vi "MAIN.vi"() -> ()   [LabVIEW 2017]
uses:
  Typedefs/Instructions.ctl
  Typedefs/State Information.ctl
  <vilib>/Utility/error.llb/DialogType.ctl
  Typedefs/Temperature Profile.ctl
  Typedefs/Status.ctl
  <vilib>/event_ctls.llb/usereventprio.ctl
  <vilib>/DAQmx/read.llb/DAQmx Read (Analog Wfm 1Chan NSamp).vi
  <vilib>/DAQmx/miscellaneous.llb/DAQmx Fill In Error Info.vi
  <vilib>/Utility/file.llb/Write To Spreadsheet File (DBL).vi
  <resource>/objmgr/daqmx.rc
panel:
  in  "Tab Control":enum32{"Settings", "Charts"}(tab)
  in  "Linkam Controller":refnum<visa-resource-name>="COM1"
  in  "Temp loop delay":u32=100
  out "Current Temperature Loop Error":errorcluster
  in  "physical channels":tag="Dev1/ai0"
  out "Slide":i32(slide) scale=15.0..1.0
  out "Voltage":waveform(dbl)(graph)
  out "Temperature":dbl(graph)
  in  "Temperature Profile":dbl[][](array[numeric])=[[20.0, 0.0], [1.0, -30.0]]
  out "Status":string
  out "Error":string
  out "Pump":u8
  out "°C":dbl
  in  "Start":bool
  in  "Hold":bool
  in  "Stop":bool
  in  "Disconnect":bool
  out "Current Ramp":i32
  out "Time (ms)":i32
  out "Loop 2 Timer":u32
  out "Loop 1 Timer":u32
  in  "Rate":dbl=1000.0 format="%0.2f"
  out "Samples":i32
  # "Rate(°C/min)"
  # "Hold (s)"
  # "Limit (°C)"
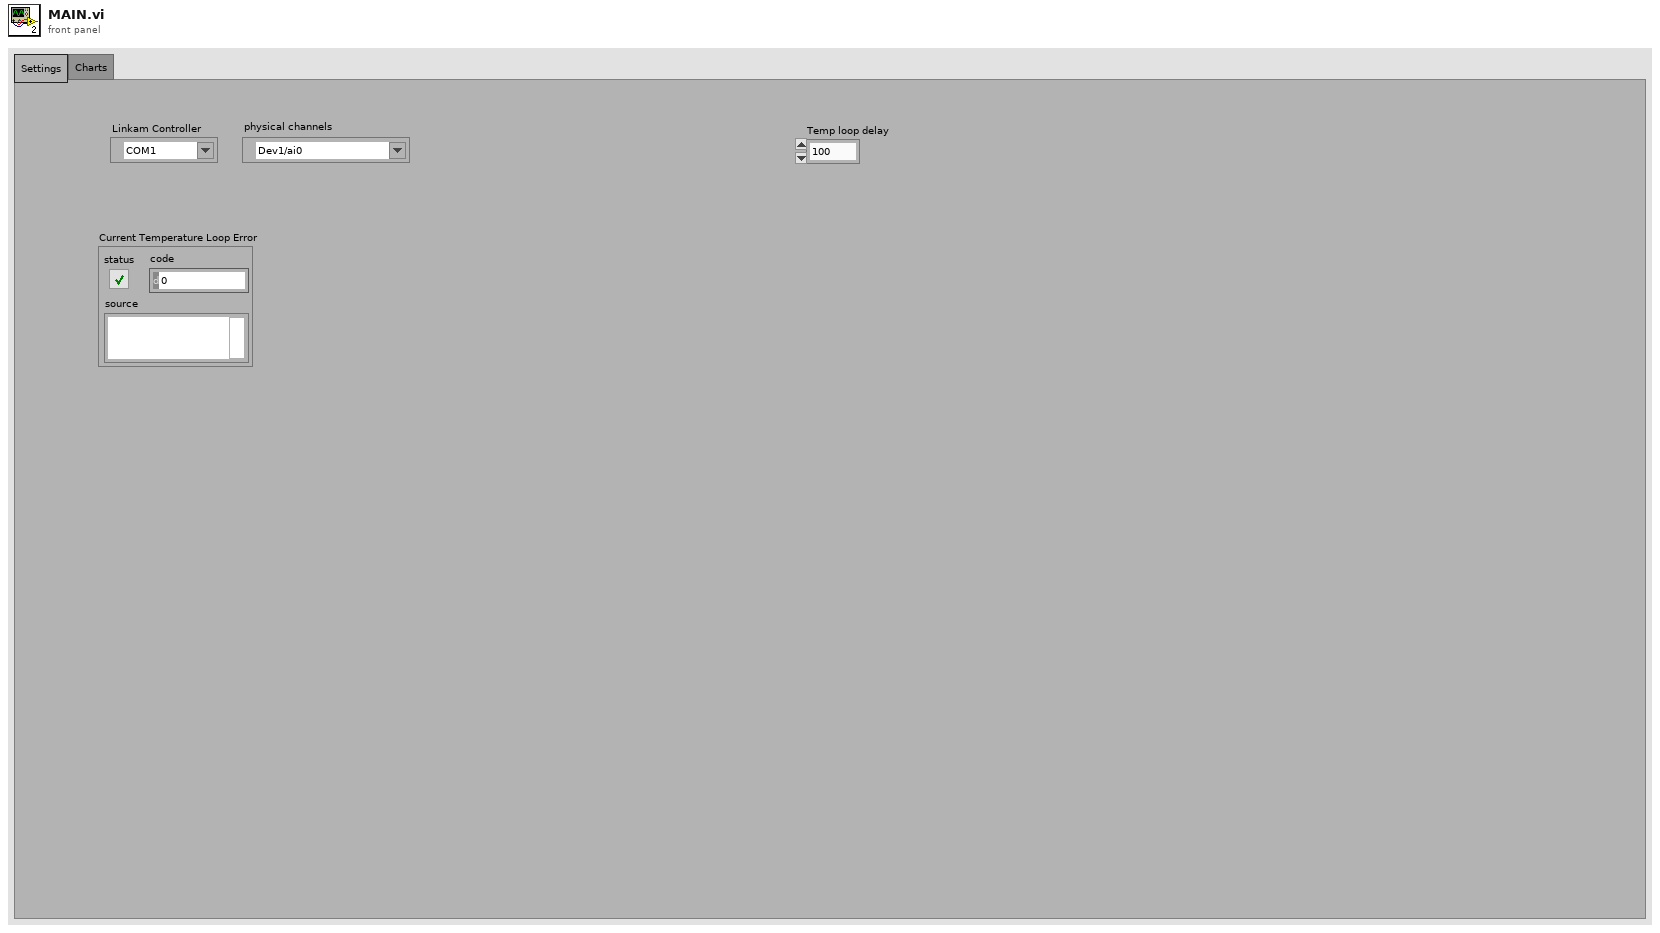
[diagram p1: front panel]
types:
  T1 = typedef "DialogType.ctl" = u16
  T2 = typedef "State Information.ctl" = cluster{"Ramp":i32, "Total Ramp":i32, "Time":i32, "Total Time":i32, "Start Time":dbl}
  T3 = typedef "Instructions.ctl" = enum16{"Idle", "Start", "Get Profile", "Go to Limit", "Hold Limit Time", "Stop", "Disconnect"}
  T4 = typedef "Temperature Profile.ctl" = enum16{"Rate", "Limit", "Hold Time"}
  T5 = typedef "Status.ctl" = enum16{"No Status", "Stopped", "Heating", "Cooling", "Limit Reached", "Holding the Limit Time", "Manual Hold"}
  T6 = typedef "usereventprio.ctl" = enum32{"high priority", "normal priority"}
  T7 = cluster{"Temperature":dbl, "Status":string, "Error":string, "Pump":u8}
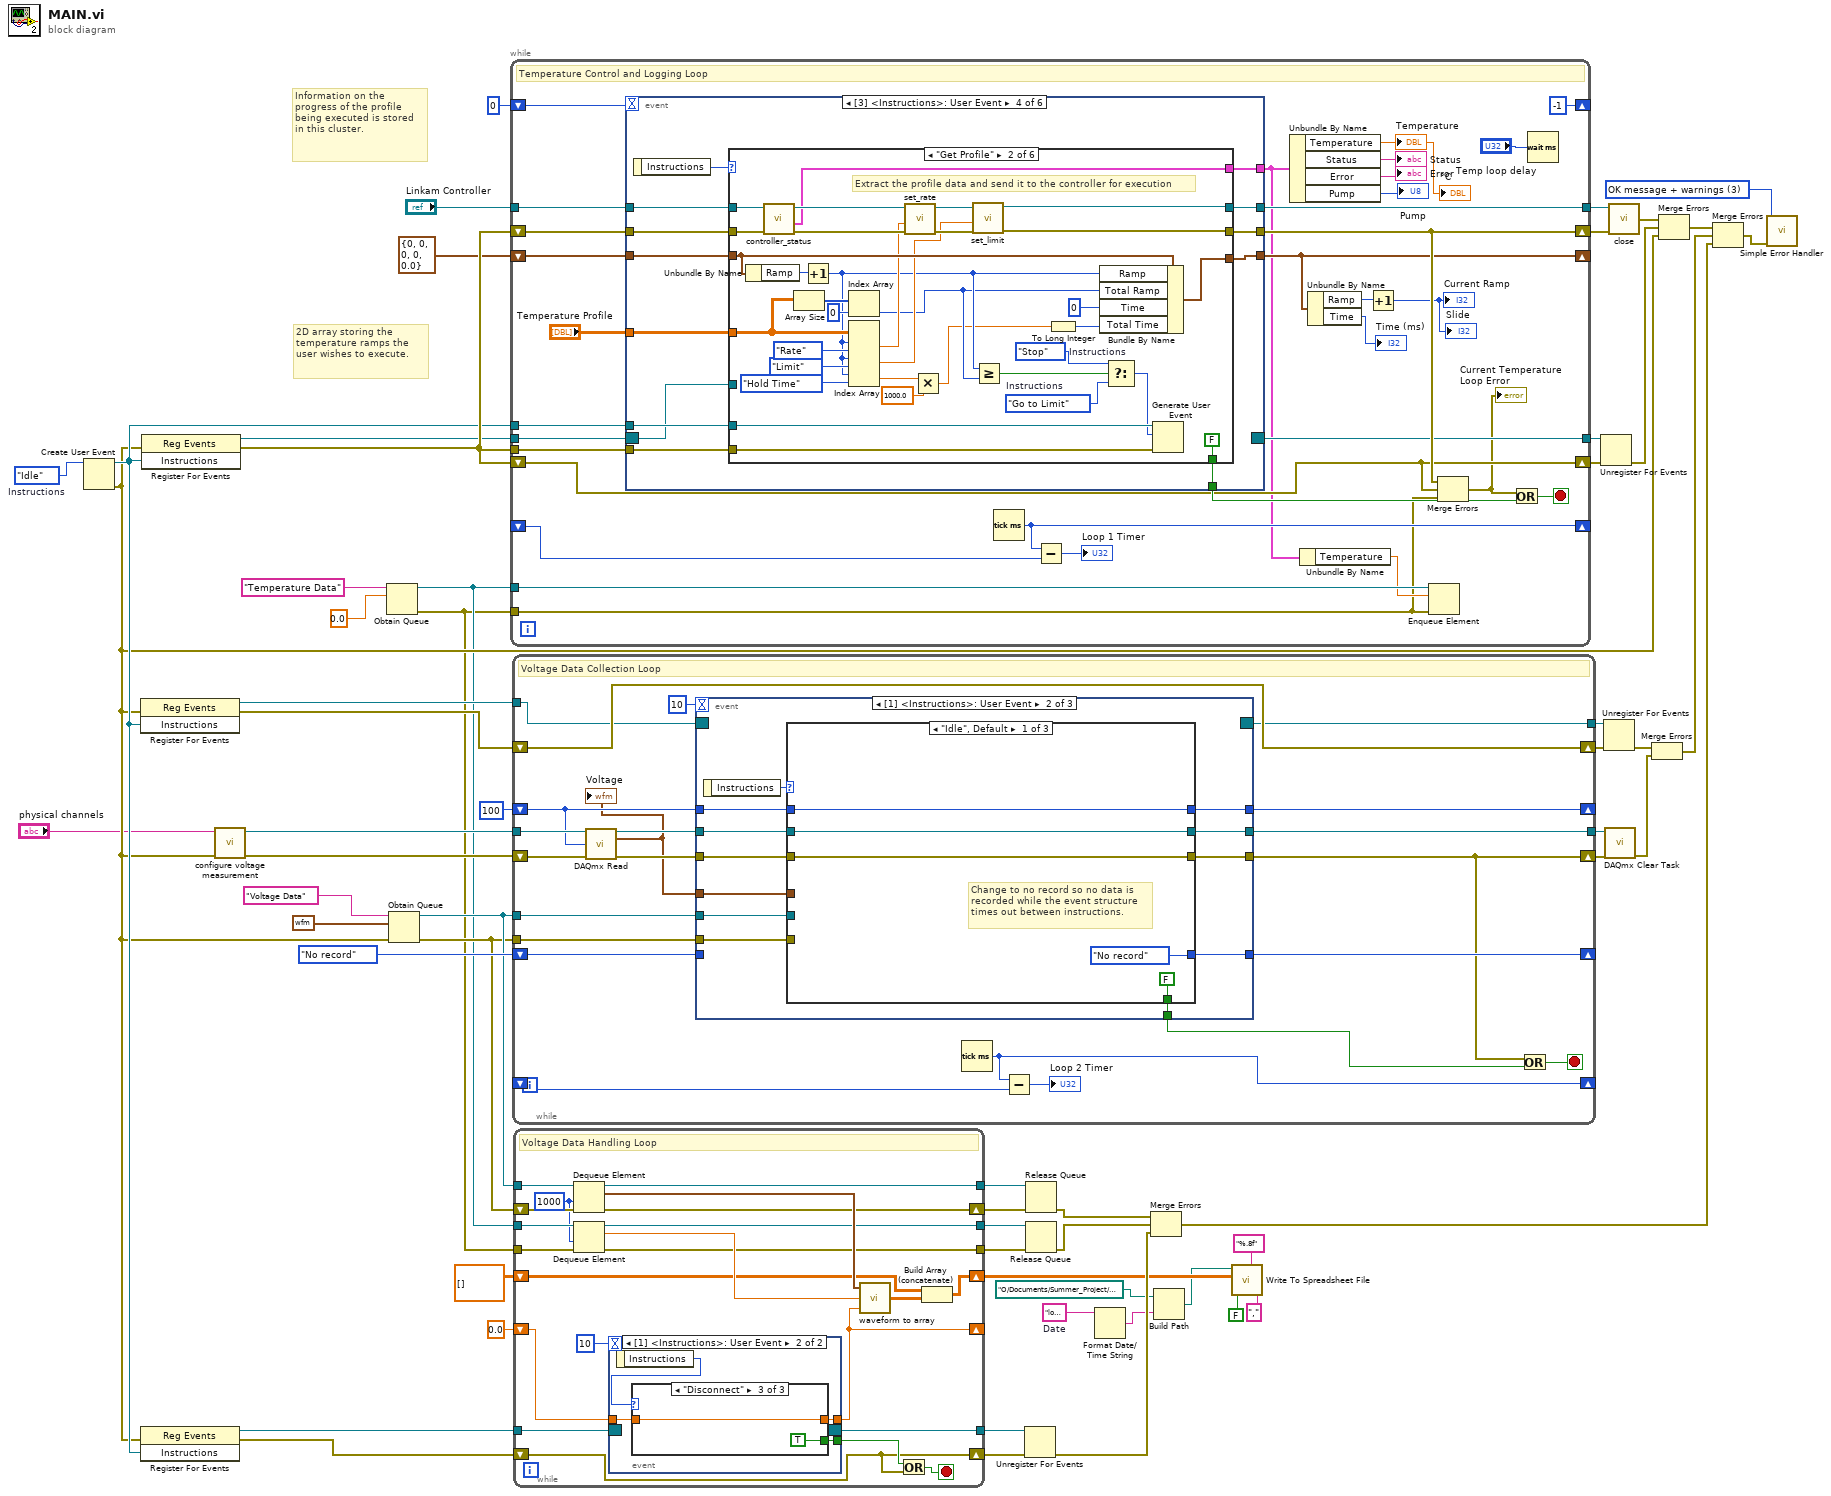
[diagram p0: block diagram]
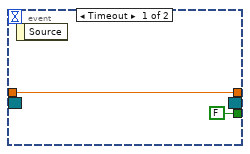
[diagram p2: hidden frame]
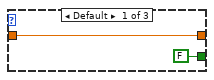
[diagram p3: hidden frame]
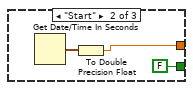
[diagram p4: hidden frame]
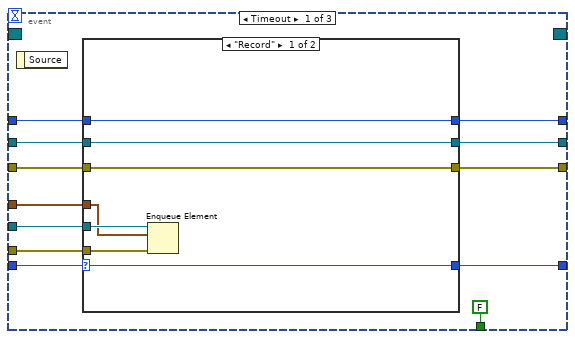
[diagram p5: hidden frame]
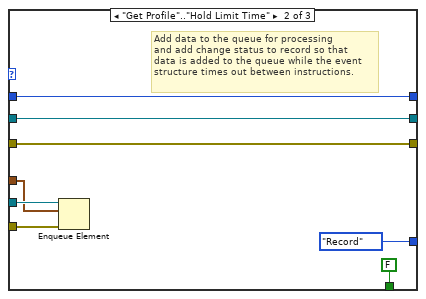
[diagram p7: hidden frame]
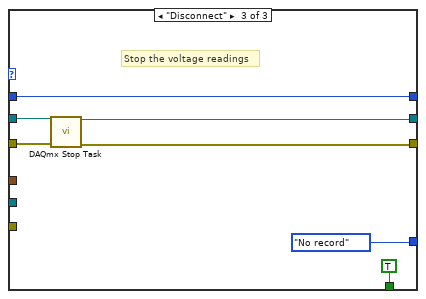
[diagram p8: hidden frame]
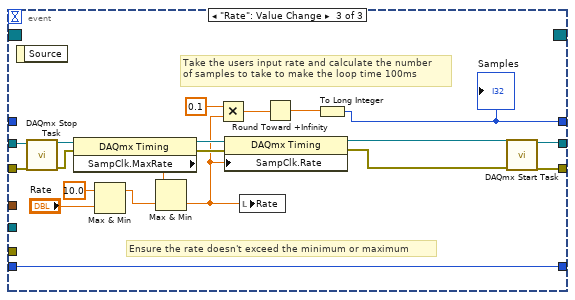
[diagram p9: hidden frame]
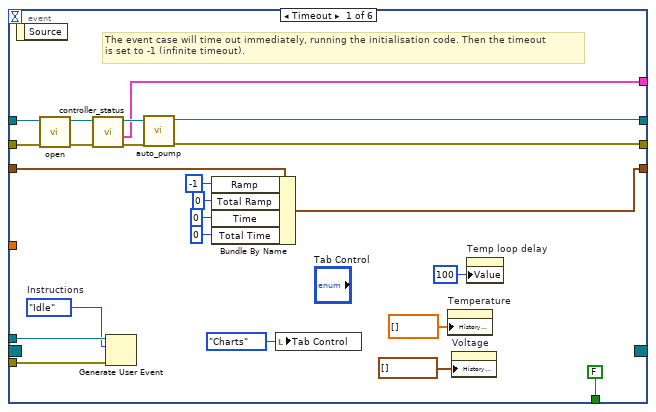
[diagram p10: hidden frame]
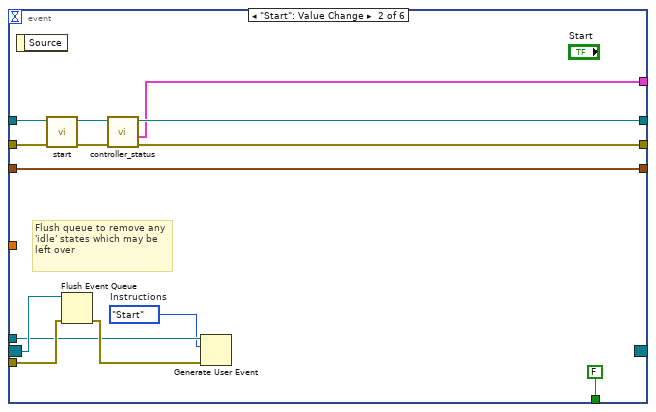
[diagram p11: hidden frame]
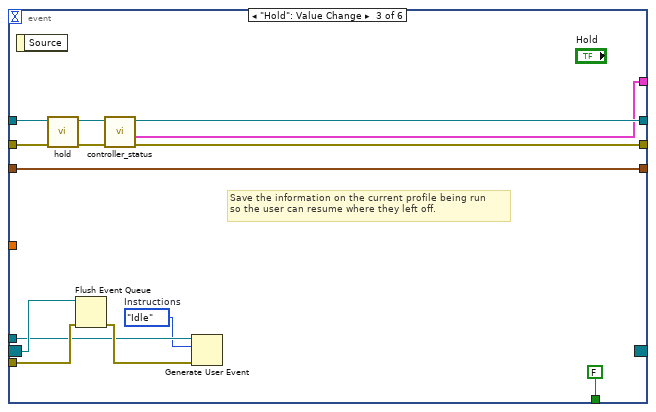
[diagram p12: hidden frame]
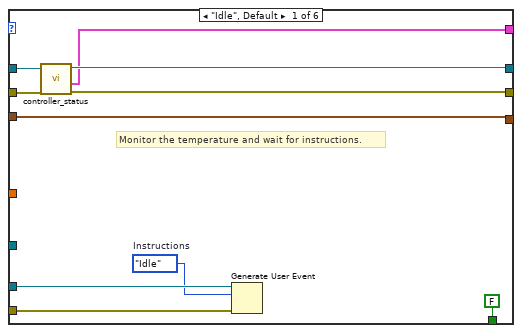
[diagram p13: hidden frame]
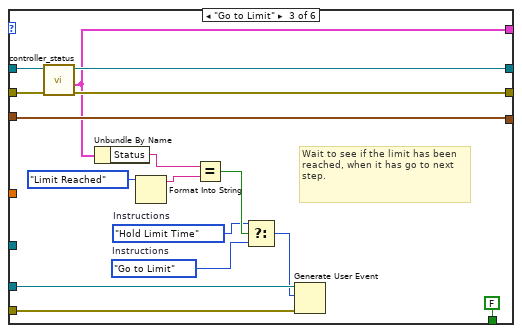
[diagram p14: hidden frame]
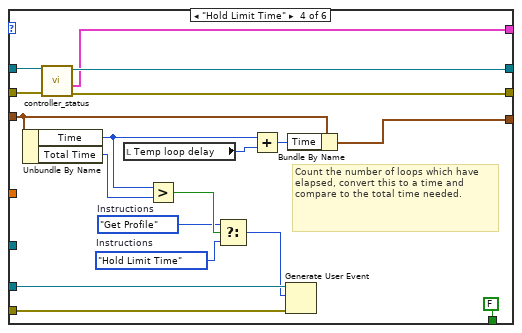
[diagram p15: hidden frame]
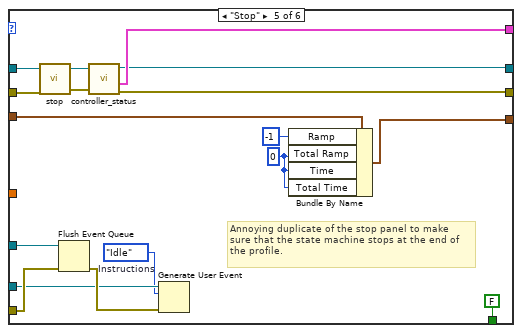
[diagram p16: hidden frame]
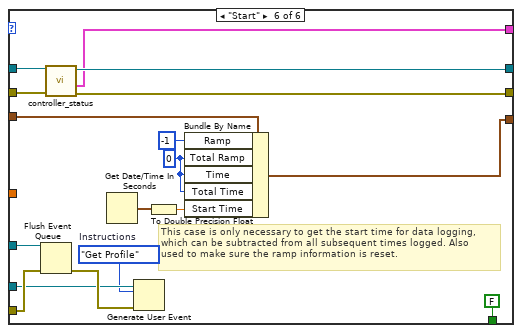
[diagram p17: hidden frame]
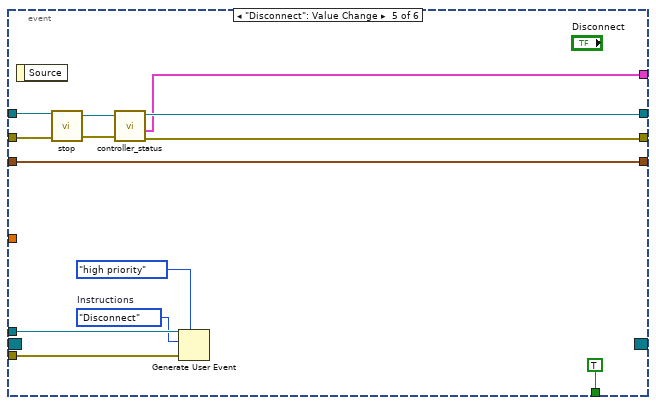
[diagram p18: hidden frame]
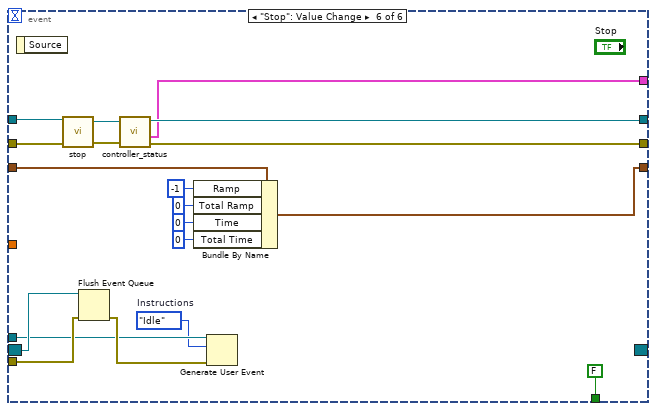
[diagram p19: hidden frame]
diagram:
  w4 = "log_%d_%m_%H%M.csv"  # Date
  w24 = T1 3 items=["no dialog", "OK message", "continue or stop message", "OK message + warnings", "continue/stop + warnings"] ("type of dialog (OK msg:1)")
  w59 = Instructions."Idle"  # Instructions
  # "Information on the progress of the profile being executed is stored in this cluster."
  # "2D array storing the temperature ramps the user wishes to execute."
  n1 = Create User Event(user event datatype=w59) -> (user event=w41:refnum<user-event>, error out=w32:errorcluster)  [unwired: 1 in]
  n2 = register-events(error in=w32, w41) -> (reference out=w52:refnum<event-registration>, error out=w49:errorcluster)  [unwired: 1 in]
  n3 = register-events(error in=w32, w41) -> (reference out=w40:refnum<event-registration>, error out=w37:errorcluster)  [unwired: 1 in]
  n4 = register-events(error in=w32, w41) -> (reference out=w60:refnum<event-registration>, error out=w61:errorcluster)  [unwired: 1 in]
  n5 = call "configure voltage measurement.vi"("error in (no error)"=w32, "physical channels"="physical channels") -> ("error out"=w46:errorcluster, "Refnum out"=w47:refnum<k21>)  [unwired: 8 in]
  n6 = Obtain Queue(name (unnamed)="Temperature Data", element data type=0.0 ("Temperature")) -> (queue out=w18:refnum<queue>, error out=w17:errorcluster)  [unwired: 3 in, 1 out]
  n7 = Obtain Queue(name (unnamed)="Voltage Data", element data type=waveform(dbl) {"t0"=timestamp(0 s since 1904-01-01), "dt"=1.0, "Y"=[]} ("data"), error in (no error)=w32) -> (queue out=w39:refnum<queue>, error out=w38:errorcluster)  [unwired: 2 in, 1 out]
  n8 = while {
    tunnel: w60 -> [w92]
    tunnel: [w91] -> w58
    shift-right: [w76] -> w57
    shift-left: w61 -> [w76]
    tunnel: "Linkam Controller" -> [w88]
    tunnel: [w86] -> w55
    shift-right: [w93] -> w54
    shift-left: w61 -> [w87]
    tunnel: w41 -> [w85]
    shift-right: [w74] -> _
    shift-left: T2 {"Ramp"=0, "Total Ramp"=0, "Time"=0, "Total Time"=0, "Start Time"=0.0} ("State Information") -> [w84]
    tunnel: w61 -> [w83]
    shift-right: [-1] -> _
    shift-left: 0 -> [w71]
    shift-right: [w68] -> _
    shift-left: _ -> [w69]
    tunnel: w18 -> [w65]
    tunnel: w17 -> [w62]
    stop <- w90 stop-if-true
    # "Temperature Control and Logging Loop"
    n9 = event shown="[3] <Instructions>: User Event" {
      selector: w92 -> [_ w121 w143 w145 _ w293]
      dyn-events: [_ _ _ _ _ _] -> w91
      timeout: w71 -> [_ _ _ _ _ _]
      tunnel: [FALSE FALSE FALSE w156 TRUE FALSE] -> w89
      tunnel: w88 -> [w113 w129 w138 w155 w281 w290]
      tunnel: w87 -> [w112 w130 w137 w154 w282 w289]
      tunnel: [w106 w126 w134 w153 w278 w286] -> w86
      tunnel: [w105 w125 w133 w152 w277 w285] -> w93
      tunnel: w85 -> [w116 w120 w140 w151 w274 w292]
      tunnel: w84 -> [w100 w117 w131 w150 w275 w299]
      tunnel: [w99 w117 w131 w149 w275 w298] -> w74
      tunnel: w83 -> [w115 w123 w142 w148 w273 w300]
      tunnel: "Temperature Profile" -> [_ _ _ w147 _ _]
      tunnel: [w107 w124 w132 w146 w276 w284] -> w64
      event Timeout {
        w114 = Instructions."Idle"  # Instructions
        # "The event case will time out immediately, running the initialisation code. Then the timeout\nis set to -1 (infinite timeout)."
        n10 = event-data() -> ()  [unwired: 1 in, 1 out]
        n11 = call "open.vi"("error in (no error)"=w112, "reference"=w113) -> ("error out"=w111:errorcluster, "reference out"=w110:refnum<visa-resource-name>)  [unwired: 8 in]
        n12 = call "controller_status.vi"("error in (no error)"=w111, "VISA Refnum in"=w110) -> ("error out"=w109:errorcluster, "output cluster"=w107:T7, "VISA Refnum out"=w108:refnum<visa-resource-name>)  [unwired: 7 in]
        n13 = Generate User Event(user event=w116, event data cluster=w114, error in=w115) -> ()  [unwired: 1 in, 2 out]
        n14 = call "auto_pump.vi"("error in (no error)"=w109, "VISA Refnum in"=w108) -> ("error out"=w105:errorcluster, "VISA Refnum out"=w106:refnum<visa-resource-name>)  [unwired: 8 in]
        n15 = Bundle By Name(cluster=w100, "Ramp"=-1, "Total Ramp"=0, "Time"=0, "Total Time"=0) -> (w99:T2)
        n16 = local write "Tab Control"(enum32{"Settings", "Charts"}."Charts" ("Tab Control")) -> ()
        n17 = property on="Temperature" class="WFChart (strict)"("History Data"=dbl[] []) -> ()  [unwired: 2 in, 2 out]
        n18 = property on="Voltage" class="WFChart (strict)"("History Data"=waveform(dbl)[] []) -> ()  [unwired: 2 in, 2 out]
        n19 = property on="Temp loop delay" class="DigNum (strict)"("Value"=u32 100 ("Temp loop delay")) -> ()  [unwired: 2 in, 2 out]
      }
      event "Start": Value Change {
        w119 = Instructions."Start"  # Instructions
        # "Flush queue to remove any 'idle' states which may be left over"
        n20 = event-data() -> ()  [unwired: 1 in, 1 out]
        n21 = call "start.vi"("error in (no error)"=w130, "VISA resource name"=w129) -> ("Error out"=w127:errorcluster, "VISA resource name out"=w128:refnum<visa-resource-name>)  [unwired: 4 in]
        n22 = Flush Event Queue(0:w121, 3:w123) -> (11:w122:errorcluster)  [unwired: 4 in, 2 out]
        n23 = call "controller_status.vi"("error in (no error)"=w127, "VISA Refnum in"=w128) -> ("error out"=w125:errorcluster, "output cluster"=w124:T7, "VISA Refnum out"=w126:refnum<visa-resource-name>)  [unwired: 7 in]
        n24 = Generate User Event(user event=w120, event data cluster=w119, error in=w122) -> ()  [unwired: 1 in, 2 out]
      }
      event "Hold": Value Change {
        w139 = Instructions."Idle"  # Instructions
        # "Save the information on the current profile being run\nso the user can resume where they left off."
        n25 = event-data() -> ()  [unwired: 1 in, 1 out]
        n26 = call "hold.vi"("error in (no error)"=w137, "VISA resource name"=w138) -> ("error out"=w135:errorcluster, "VISA resource name out"=w136:refnum<visa-resource-name>)  [unwired: 4 in]
        n27 = Flush Event Queue(0:w143, 3:w142) -> (11:w141:errorcluster)  [unwired: 4 in, 2 out]
        n28 = call "controller_status.vi"("error in (no error)"=w135, "VISA Refnum in"=w136) -> ("error out"=w133:errorcluster, "output cluster"=w132:T7, "VISA Refnum out"=w134:refnum<visa-resource-name>)  [unwired: 7 in]
        n29 = Generate User Event(user event=w140, event data cluster=w139, error in=w141) -> ()  [unwired: 1 in, 2 out]
      }
      event User Event {
        n30 = event-data() -> ("Instructions"=w157:T3)  [unwired: 1 in]
        n31 = case shown="\"Get Profile\"" w157 {
          tunnel: [FALSE FALSE FALSE FALSE FALSE FALSE] -> w156
          tunnel: w155 -> [w166 w200 w216 w234 w252 w262]
          tunnel: w154 -> [w167 w201 w217 w235 w251 w263]
          tunnel: [w165 w195 w215 w233 w247 w261] -> w153
          tunnel: [w164 w194 w214 w232 w246 w260] -> w152
          tunnel: w151 -> [w161 w174 w212 w229 w241 w254]
          tunnel: w150 -> [w162 w185 w203 w224 w245 w269]
          tunnel: [w162 w183 w203 w223 w244 w264] -> w149
          tunnel: w148 -> [w160 w173 w211 w228 w243 w256]
          tunnel: w147 -> [_ w188 _ _ _ _]
          tunnel: [w158 w171 w202 w218 w248 w259] -> w146
          tunnel: w145 -> [_ _ _ _ w240 w257]
          frame "Idle", Default {
            w159 = Instructions."Idle"  # Instructions
            # "Monitor the temperature and wait for instructions."
            n32 = call "controller_status.vi"("error in (no error)"=w167, "VISA Refnum in"=w166) -> ("error out"=w164:errorcluster, "output cluster"=w158:T7, "VISA Refnum out"=w165:refnum<visa-resource-name>)  [unwired: 7 in]
            n33 = Generate User Event(user event=w161, event data cluster=w159, error in=w160) -> ()  [unwired: 1 in, 2 out]
          }
          frame "Get Profile" {
            w176 = Instructions."Stop"  # Instructions
            w175 = Instructions."Go to Limit"  # Instructions
            # "Extract the profile data and send it to the controller for execution"
            n34 = Unbundle By Name(w185) -> ("Ramp"=w192:i32)
            n35 = call "controller_status.vi"("error in (no error)"=w201, "VISA Refnum in"=w200) -> ("error out"=w198:errorcluster, "output cluster"=w171:T7, "VISA Refnum out"=w199:refnum<visa-resource-name>)  [unwired: 7 in]
            n36 = Array Size(array=w188) -> (size(s)=w187:i32[])
            n37 = Increment(x=w192) -> (x+1=w179:i32)
            n38 = Index Array(array=w187, index=0) -> (element=w178:i32)
            n39 = Index Array(array=w188, index (row) #1=w179, index (col) #1=Temperature_Profile."Rate" ("Enum"), index (row) #2=w179, index (col) #2=Temperature_Profile."Limit" ("Enum"), index (row) #3=w179, index (col) #3=Temperature_Profile."Hold Time" ("Enum")) -> (element #1=w181:dbl, element #2=w180:dbl, element #3=w170:dbl)
            n40 = call "set_rate.vi"("error in (no error)"=w198, "Set Rate"=w181, "VISA resource name in"=w199) -> ("error out"=w196:errorcluster, "VISA resource name out"=w197:refnum<visa-resource-name>)  [unwired: 3 in]
            n41 = Multiply(x=w170, y=1000.0) -> (x*y=w168:dbl)
            n42 = call "set_limit.vi"("error in (no error)"=w196, "Set Temperature"=w180, "VISA resource name"=w197) -> ("error out"=w194:errorcluster, "VISA resource name out"=w195:refnum<visa-resource-name>)  [unwired: 3 in]
            n43 = Greater Or Equal?(x=w179, y=w178) -> (x >= y?=w177:bool)
            n44 = To Long Integer(number=w168) -> (32bit integer=w169:i32)
            n45 = Bundle By Name(cluster=w185, "Ramp"=w179, "Total Ramp"=w178, "Time"=0, "Total Time"=w169) -> (w183:T2)
            n46 = Select(t=w176, s=w177, f=w175) -> (s? t:f=w172:T3)
            n47 = Generate User Event(user event=w174, event data cluster=w172, error in=w173) -> ()  [unwired: 1 in, 2 out]
          }
          frame "Go to Limit" {
            w205 = Instructions."Go to Limit"  # Instructions
            w206 = Instructions."Hold Limit Time"  # Instructions
            # "Wait to see if the limit has been reached, when it has go to next step."
            n48 = call "controller_status.vi"("error in (no error)"=w217, "VISA Refnum in"=w216) -> ("error out"=w214:errorcluster, "output cluster"=w202:T7, "VISA Refnum out"=w215:refnum<visa-resource-name>)  [unwired: 7 in]
            n49 = Unbundle By Name(w202) -> ("Status"=w209:string)
            n50 = Format Into String(Status."Limit Reached" ("Enum")) -> (resulting string=w208:string)  [unwired: 3 in, 1 out]
            n51 = Equal?(x=w209, y=w208) -> (x = y?=w207:bool)
            n52 = Select(t=w206, s=w207, f=w205) -> (s? t:f=w204:T3)
            n53 = Generate User Event(user event=w212, event data cluster=w204, error in=w211) -> ()  [unwired: 1 in, 2 out]
          }
          frame "Hold Limit Time" {
            w225 = Instructions."Hold Limit Time"  # Instructions
            w226 = Instructions."Get Profile"  # Instructions
            # "Count the number of loops which have elapsed, convert this to a time and compare to the total time needed."
            n54 = Unbundle By Name(w224) -> ("Time"=w222:i32, "Total Time"=w230:i32)
            n55 = call "controller_status.vi"("error in (no error)"=w235, "VISA Refnum in"=w234) -> ("error out"=w232:errorcluster, "output cluster"=w218:T7, "VISA Refnum out"=w233:refnum<visa-resource-name>)  [unwired: 7 in]
            n56 = local read "Temp loop delay"() -> (w220:u32)
            n57 = Greater?(x=w222, y=w230) -> (0:w227:bool)
            n58 = Select(t=w226, s=w227, f=w225) -> (s? t:f=w221:T3)
            n59 = Add(x=w222, y=w220) -> (x+y=w219:u32)
            n60 = Generate User Event(user event=w229, event data cluster=w221, error in=w228) -> ()  [unwired: 1 in, 2 out]
            n61 = Bundle By Name(cluster=w224, "Time"=w219) -> (w223:T2)
          }
          frame "Stop" {
            w236 = 0 ("Total Ramp")
            w239 = Instructions."Idle"  # Instructions
            # "Annoying duplicate of the stop panel to make\nsure that the state machine stops at the end of\nthe profile."
            n62 = call "stop.vi"("VISA resource name"=w252, "error in (no error)"=w251) -> ("VISA resource name out"=w249:refnum<visa-resource-name>, "Error out"=w250:errorcluster)  [unwired: 6 in]
            n63 = Flush Event Queue(0:w240, 3:w243) -> (11:w242:errorcluster)  [unwired: 4 in, 2 out]
            n64 = call "controller_status.vi"("error in (no error)"=w250, "VISA Refnum in"=w249) -> ("error out"=w246:errorcluster, "output cluster"=w248:T7, "VISA Refnum out"=w247:refnum<visa-resource-name>)  [unwired: 7 in]
            n65 = Generate User Event(user event=w241, event data cluster=w239, error in=w242) -> ()  [unwired: 1 in, 2 out]
            n66 = Bundle By Name(cluster=w245, "Ramp"=-1, "Total Ramp"=w236, "Time"=w236, "Total Time"=w236) -> (w244:T2)
          }
          frame "Start" {
            w253 = Instructions."Get Profile"  # Instructions
            w265 = 0 ("Total Ramp")
            # "This case is only necessary to get the start time for data logging,\nwhich can be subtracted from all subsequent times logged. Also\nused to make sure the ramp information is reset."
            n67 = Flush Event Queue(0:w257, 3:w256) -> (11:w255:errorcluster)  [unwired: 4 in, 2 out]
            n68 = call "controller_status.vi"("error in (no error)"=w263, "VISA Refnum in"=w262) -> ("error out"=w260:errorcluster, "output cluster"=w259:T7, "VISA Refnum out"=w261:refnum<visa-resource-name>)  [unwired: 7 in]
            n69 = Get Date/Time In Seconds() -> (seconds since 1Jan1904=w267:timestamp)
            n70 = Generate User Event(user event=w254, event data cluster=w253, error in=w255) -> ()  [unwired: 1 in, 2 out]
            n71 = To Double Precision Float(number=w267) -> (double precision float=w268:dbl)
            n72 = Bundle By Name(cluster=w269, "Ramp"=-1, "Total Ramp"=w265, "Time"=w265, "Total Time"=w265, "Start Time"=w268) -> (w264:T2)
          }
        }
      }
      event "Disconnect": Value Change {
        w271 = Instructions."Disconnect"  # Instructions
        n73 = event-data() -> ()  [unwired: 1 in, 1 out]
        n74 = call "stop.vi"("VISA resource name"=w281, "error in (no error)"=w282) -> ("VISA resource name out"=w280:refnum<visa-resource-name>, "Error out"=w279:errorcluster)  [unwired: 6 in]
        n75 = call "controller_status.vi"("error in (no error)"=w279, "VISA Refnum in"=w280) -> ("error out"=w277:errorcluster, "output cluster"=w276:T7, "VISA Refnum out"=w278:refnum<visa-resource-name>)  [unwired: 7 in]
        n76 = Generate User Event(priority (normal)=usereventprio."high priority", user event=w274, event data cluster=w271, error in=w273) -> ()  [unwired: 2 out]
      }
      event "Stop": Value Change {
        w291 = Instructions."Idle"  # Instructions
        n77 = event-data() -> ()  [unwired: 1 in, 1 out]
        n78 = call "stop.vi"("VISA resource name"=w290, "error in (no error)"=w289) -> ("VISA resource name out"=w287:refnum<visa-resource-name>, "Error out"=w288:errorcluster)  [unwired: 6 in]
        n79 = Flush Event Queue(0:w293, 3:w300) -> (11:w301:errorcluster)  [unwired: 4 in, 2 out]
        n80 = call "controller_status.vi"("error in (no error)"=w288, "VISA Refnum in"=w287) -> ("error out"=w285:errorcluster, "output cluster"=w284:T7, "VISA Refnum out"=w286:refnum<visa-resource-name>)  [unwired: 7 in]
        n81 = Bundle By Name(cluster=w299, "Ramp"=-1, "Total Ramp"=0, "Time"=0, "Total Time"=0) -> (w298:T2)
        n82 = Generate User Event(user event=w292, event data cluster=w291, error in=w301) -> ()  [unwired: 1 in, 2 out]
      }
    }
    n83 = Tick Count (ms)() -> (millisecond timer value=w68:u32)
    n84 = Subtract(x=w68, y=w69) -> (x-y=→"Loop 1 Timer":u32)
    n85 = Unbundle By Name(w64) -> ("Temperature"=→"Temperature" →"°C":dbl, "Status"=→"Status":string, "Error"=→"Error":string, "Pump"=→"Pump":u8)
    n86 = Unbundle By Name(w64) -> ("Temperature"=w63:dbl)
    n87 = Unbundle By Name(w74) -> ("Ramp"=w72:i32, "Time"=→"Time (ms)":i32)
    n88 = Increment(x=w72) -> (x+1=→"Current Ramp" →"Slide":i32)
    n89 = Enqueue Element(queue=w65, element=w63, error in (no error)=w62) -> ()  [unwired: 1 in, 3 out]
    n90 = Merge Errors(w93, w76, w62) -> (w75:errorcluster)
    "Current Temperature Loop Error" <- w75
    n91 = Or(x=w75, y=w89) -> (x .or. y?=w90:bool)
    n92 = Wait (ms)(milliseconds to wait="Temp loop delay") -> ()  [unwired: 1 out]
  }
  n93 = while {
    tunnel: w52 -> [w321]
    tunnel: [w322] -> w51
    shift-right: [w317] -> _
    shift-left: _ -> [w316]
    shift-right: [w309] -> _
    shift-left: enum16{"Record", "No record"}."No record" -> [w314]
    tunnel: w47 -> [w313]
    tunnel: [w308] -> w44
    shift-right: [w307] -> _
    shift-left: 100 ("Samples Read") -> [w303]
    tunnel: w39 -> [w306]
    tunnel: w38 -> [w305]
    shift-right: [w323] -> w45
    shift-left: w49 -> [w323]
    shift-right: [w304] -> w43
    shift-left: w46 -> [w312]
    stop <- w320 stop-if-true
    # "Voltage Data Collection Loop"
    n94 = call-poly <vilib>:"DAQmx Read.vi"("task/channels in"=w313, "number of samples per channel"=w303, "error in"=w312) -> ("task out"=w311:refnum<k21>, "data"=w302:waveform(dbl), "error out"=w310:errorcluster)  [unwired: 10 in]
    "Voltage" <- w302
    n95 = event shown="[1] <Instructions>: User Event" {
      selector: w321 -> [_ _ _]
      dyn-events: [_ _ _] -> w322
      timeout: 10 -> [_ _ _]
      tunnel: [FALSE w357 _] -> w319
      tunnel: w314 -> [w334 _ w394]
      tunnel: w311 -> [w330 w350 w398]
      tunnel: w310 -> [w328 w348 w397]
      tunnel: [w324 w356 w394] -> w309
      tunnel: [w327 w347 w396] -> w304
      tunnel: [w329 w349 w395] -> w308
      tunnel: [w325 w351 w384] -> w307
      tunnel: w303 -> [w326 w352 _]
      tunnel: w306 -> [w333 w355 _]
      tunnel: w305 -> [w332 w354 _]
      tunnel: w302 -> [w331 w353 _]
      event Timeout {
        n96 = event-data() -> ()  [unwired: 1 in, 1 out]
        n97 = case shown="\"Record\"" w334 {
          selector: w334 -> [w337 w343]
          tunnel: w333 -> [w339 _]
          tunnel: w332 -> [w338 _]
          tunnel: w331 -> [w336 _]
          tunnel: [w341 w346] -> w329
          tunnel: w330 -> [w341 w346]
          tunnel: w328 -> [w340 w345]
          tunnel: [w340 w345] -> w327
          tunnel: w326 -> [w342 w344]
          tunnel: [w342 w344] -> w325
          tunnel: [w337 w343] -> w324
          frame "Record" {
            n98 = Enqueue Element(queue=w339, element=w336, error in (no error)=w338) -> ()  [unwired: 1 in, 3 out]
          }
          frame "No record", Default {
          }
        }
      }
      event User Event {
        n99 = event-data() -> ("Instructions"=w358:T3)  [unwired: 1 in]
        n100 = case shown="\"Idle\", Default" w358 {
          tunnel: [FALSE FALSE TRUE] -> w357
          tunnel: [enum16{"Record", "No record"}."No record" enum16{"Record", "No record"}."Record" enum16{"Record", "No record"}."No record"] -> w356
          tunnel: w355 -> [_ w369 _]
          tunnel: w354 -> [_ w368 _]
          tunnel: w353 -> [_ w364 _]
          tunnel: w352 -> [w361 w367 w376]
          tunnel: [w361 w367 w376] -> w351
          tunnel: w350 -> [w360 w366 w375]
          tunnel: [w360 w366 w373] -> w349
          tunnel: w348 -> [w359 w365 w374]
          tunnel: [w359 w365 w372] -> w347
          frame "Idle", Default {
            # "Change to no record so no data is\nrecorded while the event structure\ntimes out between instructions."
          }
          frame "Get Profile".."Hold Limit Time" {
            # "Add data to the queue for processing\nand add change status to record so that\ndata is added to the queue while the event\nstructure times out between instructions."
            n101 = Enqueue Element(queue=w369, element=w364, error in (no error)=w368) -> ()  [unwired: 1 in, 3 out]
          }
          frame "Disconnect" {
            # "Stop the voltage readings"
            n102 = call <vilib>:"DAQmx Stop Task.vi"("task/channels in"=w375, "error in"=w374) -> ("task out"=w373:refnum<k21>, "error out"=w372:errorcluster)  [unwired: 12 in]
          }
        }
      }
      event "Rate": Value Change {
        # "Ensure the rate doesn't exceed the minimum or maximum"
        # "Take the users input rate and calculate the number\nof samples to take to make the loop time 100ms"
        n103 = event-data() -> ()  [unwired: 1 in, 1 out]
        n104 = call <vilib>:"DAQmx Stop Task.vi"("task/channels in"=w398, "error in"=w397) -> ("task out"=w392:refnum<k21>, "error out"=w393:errorcluster)  [unwired: 12 in]
        n105 = property class="DAQmx Timing"(reference=w392, error in=w393) -> (reference out=w390:refnum<k21>, error out=w389:errorcluster, "SampClk.MaxRate"=w391:dbl)
        n106 = Max & Min(x=10.0, y="Rate") -> (max(x,y)=w382:dbl)  [unwired: 1 out]
        n107 = Max & Min(x=w391, y=w382) -> (min(x,y)=w386:dbl)  [unwired: 1 out]
        n108 = Multiply(x=0.1, y=w386) -> (x*y=w380:dbl)
        n109 = property class="DAQmx Timing"(reference=w390, error in=w389, "SampClk.Rate"=w386) -> (reference out=w388:refnum<k21>, error out=w387:errorcluster)
        n110 = local write "Rate"(w386) -> ()
        n111 = Round Toward +Infinity(x=w380) -> (ceil(x): smallest int >= x=w379:dbl)
        n112 = To Long Integer(number=w379) -> (32bit integer=w384:i32)
        "Samples" <- w384
        n113 = call <vilib>:"DAQmx Start Task.vi"("task/channels in"=w388, "error in"=w387) -> ("task out"=w395:refnum<k21>, "error out"=w396:errorcluster)  [unwired: 12 in]
      }
    }
    n114 = Tick Count (ms)() -> (millisecond timer value=w317:u32)
    n115 = Subtract(x=w317, y=w316) -> (x-y=→"Loop 2 Timer":u32)
    n116 = Or(x=w304, y=w319) -> (x .or. y?=w320:bool)
  }
  n117 = while {
    tunnel: w40 -> [w410]
    tunnel: w39 -> [w420]
    shift-right: [w400] -> w35
    shift-left: w37 -> [w400]
    shift-right: [w414] -> w36
    shift-left: w38 -> [w419]
    tunnel: [w407] -> w19
    tunnel: w18 -> [w418]
    tunnel: w17 -> [w417]
    shift-right: [w408] -> _
    shift-left: 0.0 -> [w409]
    tunnel: [w413] -> w15
    tunnel: [w412] -> w14
    tunnel: [w411] -> w13
    shift-right: [w403] -> w8
    shift-left: dbl[][] [] -> [w402]
    stop <- w399 stop-if-true
    w405 = 1000 ("timeout in ms (-1)")
    # "Voltage Data Handling Loop"
    n118 = Dequeue Element(queue=w420, timeout in ms (-1)=w405, error in (no error)=w419) -> (queue out=w413:refnum<queue>, element=w415:waveform(dbl), error out=w414:errorcluster)  [unwired: 1 out]
    n119 = Dequeue Element(queue=w418, timeout in ms (-1)=w405, error in (no error)=w417) -> (queue out=w412:refnum<queue>, element=w416:dbl, error out=w411:errorcluster)  [unwired: 1 out]
    n120 = event shown="[1] <Instructions>: User Event" {
      selector: w410 -> [_ _]
      dyn-events: [_ _] -> w407
      timeout: 10 -> [_ _]
      tunnel: w409 -> [w421 w425]
      tunnel: [w421 w424] -> w408
      tunnel: [FALSE w423] -> w401
      event Timeout {
        n121 = event-data() -> ()  [unwired: 1 in, 1 out]
      }
      event User Event {
        n122 = event-data() -> ("Instructions"=w426:T3)  [unwired: 1 in]
        n123 = case shown="\"Disconnect\"" w426 {
          tunnel: [FALSE FALSE TRUE] -> w423
          tunnel: [w427 w429 w432] -> w424
          tunnel: w425 -> [w427 _ w432]
          frame Default {
          }
          frame "Start" {
            n124 = Get Date/Time In Seconds() -> (seconds since 1Jan1904=w431:timestamp)
            n125 = To Double Precision Float(number=w431) -> (double precision float=w429:dbl)
          }
          frame "Disconnect" {
          }
        }
      }
    }
    n126 = call "waveform to array.vi"("Start Time"=w408, "Temperature"=w416, "Voltage Data"=w415) -> ("array"=w404:dbl[][])
    n127 = Or(x=w401, y=w400) -> (x .or. y?=w399:bool)
    n128 = Build Array (concatenate)(w402, w404) -> (w403:dbl[][])
  }
  n129 = Unregister For Events(event registration refnum=w19, error in=w35) -> (error out=w10:errorcluster)
  n130 = Release Queue(queue=w15, error in (no error)=w36) -> (error out=w12:errorcluster)  [unwired: 1 in, 2 out]
  n131 = Release Queue(queue=w14, error in (no error)=w13) -> (error out=w11:errorcluster)  [unwired: 1 in, 2 out]
  n132 = Format Date/Time String(time format string (%c)=w4) -> (date/time string=w3:string)  [unwired: 2 in]
  n133 = Merge Errors(w12, w11, w10) -> (w27:errorcluster)
  n134 = Build Path(base path=path "O:/Documents/Summer_Project/Data", name or relative path=w3) -> (appended path=w2:path)
  n135 = call-poly <vilib>:"Write To Spreadsheet File.vi"("delimiter (\\t)"="," ("delimiter (\\t)"), "format (%.3f)"="%.8f", "append to file? (new file:F)"=FALSE, "2D data"=w8, "file path (dialog if empty)"=w2) -> ()  [unwired: 3 in, 1 out]
  n136 = Unregister For Events(event registration refnum=w58, error in=w57) -> (error out=w33:errorcluster)
  n137 = Unregister For Events(event registration refnum=w51, error in=w45) -> (error out=w31:errorcluster)
  n138 = call <vilib>:"DAQmx Clear Task.vi"("task in"=w44, "error in"=w43) -> ("error out"=w30:errorcluster)  [unwired: 13 in]
  n139 = call "close.vi"("Error in"=w54, "VISA resource name"=w55) -> ("Error out"=w34:errorcluster)  [unwired: 2 in]
  n140 = Merge Errors(w31, w30) -> (w28:errorcluster)
  n141 = Merge Errors(w34, w33, w32) -> (w29:errorcluster)
  n142 = Merge Errors(w29, w28, w27) -> (w25:errorcluster)
  n143 = call <vilib>:"Simple Error Handler.vi"("type of dialog (OK msg:1)"=w24, "error in (no error)"=w25) -> ()  [unwired: 3 in, 5 out]
